vi "QDC_Histogram.vi"(3 "Hist array in":u16[][](array[numeric]), 5 "Data In":T1[](array[typedef])) -> (1 "Hist array out":u16[][](array[numeric]))   [LabVIEW 2014]
uses:
  QDCDataCluster.ctl
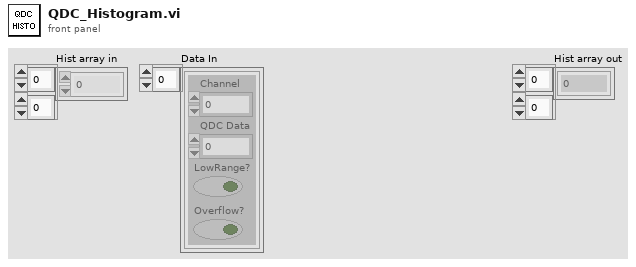
[diagram p1: front panel]
types:
  T1 = typedef "QDCDataCluster.ctl" = cluster{"Channel":u8, "QDC Data":sgl, "LowRange?":bool, "Overflow?":bool}
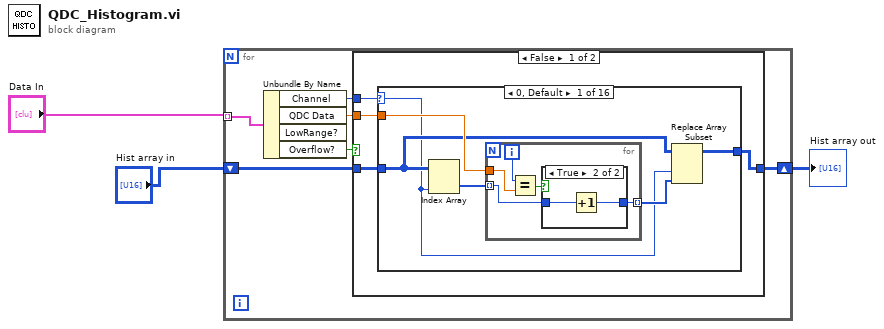
[diagram p0: block diagram]
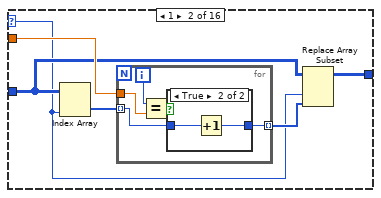
[diagram p3: hidden frame]
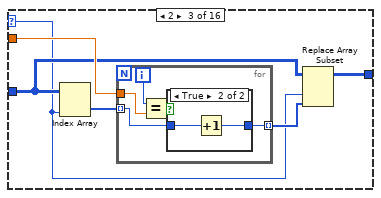
[diagram p5: hidden frame]
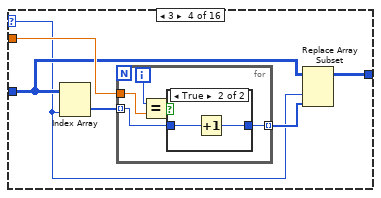
[diagram p7: hidden frame]
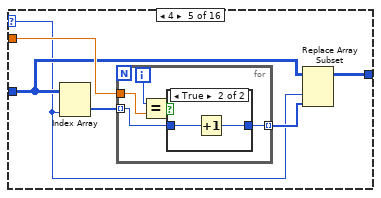
[diagram p9: hidden frame]
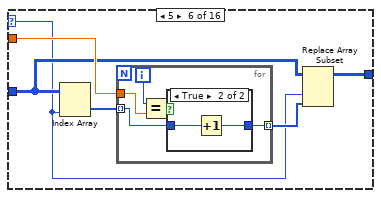
[diagram p11: hidden frame]
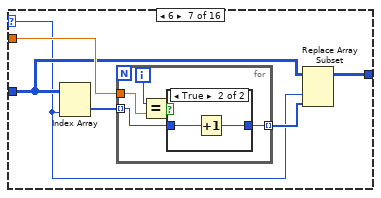
[diagram p13: hidden frame]
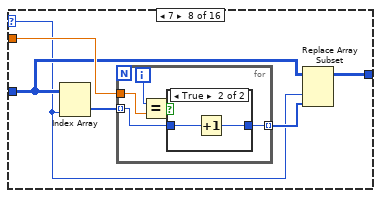
[diagram p15: hidden frame]
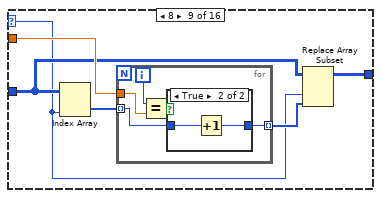
[diagram p17: hidden frame]
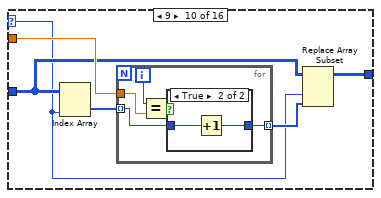
[diagram p19: hidden frame]
diagram:
  n1 = for {
    tunnel: "Data In" -> [w9] mode=indexing
    shift-right: [w5] -> w2
    shift-left: "Hist array in" -> [w6]
    n2 = Unbundle By Name(w9) -> ("Channel"=w8:u8, "QDC Data"=w7:sgl, "Overflow?"=w4:bool)  [unwired: 1 out]
    n3 = case shown="False" w4 {
      tunnel: w8 -> [w13 _]
      tunnel: w7 -> [w12 _]
      tunnel: w6 -> [w11 w238]
      tunnel: [w10 w238] -> w5
      frame False {
        n4 = case shown="0, Default" w13 {
          selector: w13 -> [w15 w29 w43 w57 w71 w85 w99 w113 w127 w141 w155 w169 w183 w197 w211 w225]
          tunnel: w12 -> [w18 w32 w46 w60 w74 w88 w102 w116 w130 w144 w158 w172 w186 w200 w214 w228]
          tunnel: w11 -> [w17 w31 w45 w59 w73 w87 w101 w115 w129 w143 w157 w171 w185 w199 w213 w227]
          tunnel: [w14 w28 w42 w56 w70 w84 w98 w112 w126 w140 w154 w168 w182 w196 w210 w224] -> w10
          frame 0, Default {
            n5 = Index Array(array=w17, index (col)=w15) -> (element=w19:u16[])  [unwired: 1 in]
            n6 = for {
              tunnel: w19 -> [w21] mode=indexing
              tunnel: w18 -> [w22]
              tunnel: [w20] -> w16 mode=indexing
              i -> [w23]
              n7 = Equal?(x=w23, y=w22) -> (x = y?=w24:bool)
              n8 = case shown="True" w24 {
                tunnel: w21 -> [w25 w27]
                tunnel: [w25 w26] -> w20
                frame False {
                }
                frame True {
                  n9 = Increment(x=w27) -> (x+1=w26:u16)
                }
              }
            }
            n10 = Replace Array Subset(array=w17, new element=w16, index (col)=w15) -> (w14:u16[][])  [unwired: 1 in]
          }
          frame 1 {
            n11 = Index Array(array=w31, index (col)=w29) -> (element=w33:u16[])  [unwired: 1 in]
            n12 = for {
              tunnel: w33 -> [w35] mode=indexing
              tunnel: w32 -> [w36]
              tunnel: [w34] -> w30 mode=indexing
              i -> [w37]
              n13 = Equal?(x=w37, y=w36) -> (x = y?=w38:bool)
              n14 = case shown="True" w38 {
                tunnel: w35 -> [w39 w41]
                tunnel: [w39 w40] -> w34
                frame False {
                }
                frame True {
                  n15 = Increment(x=w41) -> (x+1=w40:u16)
                }
              }
            }
            n16 = Replace Array Subset(array=w31, new element=w30, index (col)=w29) -> (w28:u16[][])  [unwired: 1 in]
          }
          frame 2 {
            n17 = Index Array(array=w45, index (col)=w43) -> (element=w47:u16[])  [unwired: 1 in]
            n18 = for {
              tunnel: w47 -> [w49] mode=indexing
              tunnel: w46 -> [w50]
              tunnel: [w48] -> w44 mode=indexing
              i -> [w51]
              n19 = Equal?(x=w51, y=w50) -> (x = y?=w52:bool)
              n20 = case shown="True" w52 {
                tunnel: w49 -> [w53 w55]
                tunnel: [w53 w54] -> w48
                frame False {
                }
                frame True {
                  n21 = Increment(x=w55) -> (x+1=w54:u16)
                }
              }
            }
            n22 = Replace Array Subset(array=w45, new element=w44, index (col)=w43) -> (w42:u16[][])  [unwired: 1 in]
          }
          frame 3 {
            n23 = Index Array(array=w59, index (col)=w57) -> (element=w61:u16[])  [unwired: 1 in]
            n24 = for {
              tunnel: w61 -> [w63] mode=indexing
              tunnel: w60 -> [w64]
              tunnel: [w62] -> w58 mode=indexing
              i -> [w65]
              n25 = Equal?(x=w65, y=w64) -> (x = y?=w66:bool)
              n26 = case shown="True" w66 {
                tunnel: w63 -> [w67 w69]
                tunnel: [w67 w68] -> w62
                frame False {
                }
                frame True {
                  n27 = Increment(x=w69) -> (x+1=w68:u16)
                }
              }
            }
            n28 = Replace Array Subset(array=w59, new element=w58, index (col)=w57) -> (w56:u16[][])  [unwired: 1 in]
          }
          frame 4 {
            n29 = Index Array(array=w73, index (col)=w71) -> (element=w75:u16[])  [unwired: 1 in]
            n30 = for {
              tunnel: w75 -> [w77] mode=indexing
              tunnel: w74 -> [w78]
              tunnel: [w76] -> w72 mode=indexing
              i -> [w79]
              n31 = Equal?(x=w79, y=w78) -> (x = y?=w80:bool)
              n32 = case shown="True" w80 {
                tunnel: w77 -> [w81 w83]
                tunnel: [w81 w82] -> w76
                frame False {
                }
                frame True {
                  n33 = Increment(x=w83) -> (x+1=w82:u16)
                }
              }
            }
            n34 = Replace Array Subset(array=w73, new element=w72, index (col)=w71) -> (w70:u16[][])  [unwired: 1 in]
          }
          frame 5 {
            n35 = Index Array(array=w87, index (col)=w85) -> (element=w89:u16[])  [unwired: 1 in]
            n36 = for {
              tunnel: w89 -> [w91] mode=indexing
              tunnel: w88 -> [w92]
              tunnel: [w90] -> w86 mode=indexing
              i -> [w93]
              n37 = Equal?(x=w93, y=w92) -> (x = y?=w94:bool)
              n38 = case shown="True" w94 {
                tunnel: w91 -> [w95 w97]
                tunnel: [w95 w96] -> w90
                frame False {
                }
                frame True {
                  n39 = Increment(x=w97) -> (x+1=w96:u16)
                }
              }
            }
            n40 = Replace Array Subset(array=w87, new element=w86, index (col)=w85) -> (w84:u16[][])  [unwired: 1 in]
          }
          frame 6 {
            n41 = Index Array(array=w101, index (col)=w99) -> (element=w103:u16[])  [unwired: 1 in]
            n42 = for {
              tunnel: w103 -> [w105] mode=indexing
              tunnel: w102 -> [w106]
              tunnel: [w104] -> w100 mode=indexing
              i -> [w107]
              n43 = Equal?(x=w107, y=w106) -> (x = y?=w108:bool)
              n44 = case shown="True" w108 {
                tunnel: w105 -> [w109 w111]
                tunnel: [w109 w110] -> w104
                frame False {
                }
                frame True {
                  n45 = Increment(x=w111) -> (x+1=w110:u16)
                }
              }
            }
            n46 = Replace Array Subset(array=w101, new element=w100, index (col)=w99) -> (w98:u16[][])  [unwired: 1 in]
          }
          frame 7 {
            n47 = Index Array(array=w115, index (col)=w113) -> (element=w117:u16[])  [unwired: 1 in]
            n48 = for {
              tunnel: w117 -> [w119] mode=indexing
              tunnel: w116 -> [w120]
              tunnel: [w118] -> w114 mode=indexing
              i -> [w121]
              n49 = Equal?(x=w121, y=w120) -> (x = y?=w122:bool)
              n50 = case shown="True" w122 {
                tunnel: w119 -> [w123 w125]
                tunnel: [w123 w124] -> w118
                frame False {
                }
                frame True {
                  n51 = Increment(x=w125) -> (x+1=w124:u16)
                }
              }
            }
            n52 = Replace Array Subset(array=w115, new element=w114, index (col)=w113) -> (w112:u16[][])  [unwired: 1 in]
          }
          frame 8 {
            n53 = Index Array(array=w129, index (col)=w127) -> (element=w131:u16[])  [unwired: 1 in]
            n54 = for {
              tunnel: w131 -> [w133] mode=indexing
              tunnel: w130 -> [w134]
              tunnel: [w132] -> w128 mode=indexing
              i -> [w135]
              n55 = Equal?(x=w135, y=w134) -> (x = y?=w136:bool)
              n56 = case shown="True" w136 {
                tunnel: w133 -> [w137 w139]
                tunnel: [w137 w138] -> w132
                frame False {
                }
                frame True {
                  n57 = Increment(x=w139) -> (x+1=w138:u16)
                }
              }
            }
            n58 = Replace Array Subset(array=w129, new element=w128, index (col)=w127) -> (w126:u16[][])  [unwired: 1 in]
          }
          frame 9 {
            n59 = Index Array(array=w143, index (col)=w141) -> (element=w145:u16[])  [unwired: 1 in]
            n60 = for {
              tunnel: w145 -> [w147] mode=indexing
              tunnel: w144 -> [w148]
              tunnel: [w146] -> w142 mode=indexing
              i -> [w149]
              n61 = Equal?(x=w149, y=w148) -> (x = y?=w150:bool)
              n62 = case shown="True" w150 {
                tunnel: w147 -> [w151 w153]
                tunnel: [w151 w152] -> w146
                frame False {
                }
                frame True {
                  n63 = Increment(x=w153) -> (x+1=w152:u16)
                }
              }
            }
            n64 = Replace Array Subset(array=w143, new element=w142, index (col)=w141) -> (w140:u16[][])  [unwired: 1 in]
          }
          frame 10 {
            n65 = Index Array(array=w157, index (col)=w155) -> (element=w159:u16[])  [unwired: 1 in]
            n66 = for {
              tunnel: w159 -> [w161] mode=indexing
              tunnel: w158 -> [w162]
              tunnel: [w160] -> w156 mode=indexing
              i -> [w163]
              n67 = Equal?(x=w163, y=w162) -> (x = y?=w164:bool)
              n68 = case shown="True" w164 {
                tunnel: w161 -> [w165 w167]
                tunnel: [w165 w166] -> w160
                frame False {
                }
                frame True {
                  n69 = Increment(x=w167) -> (x+1=w166:u16)
                }
              }
            }
            n70 = Replace Array Subset(array=w157, new element=w156, index (col)=w155) -> (w154:u16[][])  [unwired: 1 in]
          }
          frame 11 {
            n71 = Index Array(array=w171, index (col)=w169) -> (element=w173:u16[])  [unwired: 1 in]
            n72 = for {
              tunnel: w173 -> [w175] mode=indexing
              tunnel: w172 -> [w176]
              tunnel: [w174] -> w170 mode=indexing
              i -> [w177]
              n73 = Equal?(x=w177, y=w176) -> (x = y?=w178:bool)
              n74 = case shown="True" w178 {
                tunnel: w175 -> [w179 w181]
                tunnel: [w179 w180] -> w174
                frame False {
                }
                frame True {
                  n75 = Increment(x=w181) -> (x+1=w180:u16)
                }
              }
            }
            n76 = Replace Array Subset(array=w171, new element=w170, index (col)=w169) -> (w168:u16[][])  [unwired: 1 in]
          }
          frame 12 {
            n77 = Index Array(array=w185, index (col)=w183) -> (element=w187:u16[])  [unwired: 1 in]
            n78 = for {
              tunnel: w187 -> [w189] mode=indexing
              tunnel: w186 -> [w190]
              tunnel: [w188] -> w184 mode=indexing
              i -> [w191]
              n79 = Equal?(x=w191, y=w190) -> (x = y?=w192:bool)
              n80 = case shown="True" w192 {
                tunnel: w189 -> [w193 w195]
                tunnel: [w193 w194] -> w188
                frame False {
                }
                frame True {
                  n81 = Increment(x=w195) -> (x+1=w194:u16)
                }
              }
            }
            n82 = Replace Array Subset(array=w185, new element=w184, index (col)=w183) -> (w182:u16[][])  [unwired: 1 in]
          }
          frame 13 {
            n83 = Index Array(array=w199, index (col)=w197) -> (element=w201:u16[])  [unwired: 1 in]
            n84 = for {
              tunnel: w201 -> [w203] mode=indexing
              tunnel: w200 -> [w204]
              tunnel: [w202] -> w198 mode=indexing
              i -> [w205]
              n85 = Equal?(x=w205, y=w204) -> (x = y?=w206:bool)
              n86 = case shown="True" w206 {
                tunnel: w203 -> [w207 w209]
                tunnel: [w207 w208] -> w202
                frame False {
                }
                frame True {
                  n87 = Increment(x=w209) -> (x+1=w208:u16)
                }
              }
            }
            n88 = Replace Array Subset(array=w199, new element=w198, index (col)=w197) -> (w196:u16[][])  [unwired: 1 in]
          }
          frame 14 {
            n89 = Index Array(array=w213, index (col)=w211) -> (element=w215:u16[])  [unwired: 1 in]
            n90 = for {
              tunnel: w215 -> [w217] mode=indexing
              tunnel: w214 -> [w218]
              tunnel: [w216] -> w212 mode=indexing
              i -> [w219]
              n91 = Equal?(x=w219, y=w218) -> (x = y?=w220:bool)
              n92 = case shown="True" w220 {
                tunnel: w217 -> [w221 w223]
                tunnel: [w221 w222] -> w216
                frame False {
                }
                frame True {
                  n93 = Increment(x=w223) -> (x+1=w222:u16)
                }
              }
            }
            n94 = Replace Array Subset(array=w213, new element=w212, index (col)=w211) -> (w210:u16[][])  [unwired: 1 in]
          }
          frame 15 {
            n95 = Index Array(array=w227, index (col)=w225) -> (element=w229:u16[])  [unwired: 1 in]
            n96 = for {
              tunnel: w229 -> [w232] mode=indexing
              tunnel: w228 -> [w230]
              tunnel: [w231] -> w226 mode=indexing
              i -> [w233]
              n97 = Equal?(x=w233, y=w230) -> (x = y?=w234:bool)
              n98 = case shown="True" w234 {
                tunnel: w232 -> [w235 w237]
                tunnel: [w235 w236] -> w231
                frame False {
                }
                frame True {
                  n99 = Increment(x=w237) -> (x+1=w236:u16)
                }
              }
            }
            n100 = Replace Array Subset(array=w227, new element=w226, index (col)=w225) -> (w224:u16[][])  [unwired: 1 in]
          }
        }
      }
      frame True {
      }
    }
  }
  "Hist array out" <- w2
